vi "read section.vi"(11 "section":string="S1") -> (3 "output cluster":T1)   [LabVIEW 2017, in "GUI.lvlib"]
uses:
  GUI.lvlib
  <vilib>/Utility/config.llb/NI_LVConfig.lvlib
panel:
  in  "PxS":T2
  in  "Px":T3
  in  "Tx":T4
  in  "TxO":T5
  in  "TxA":T6
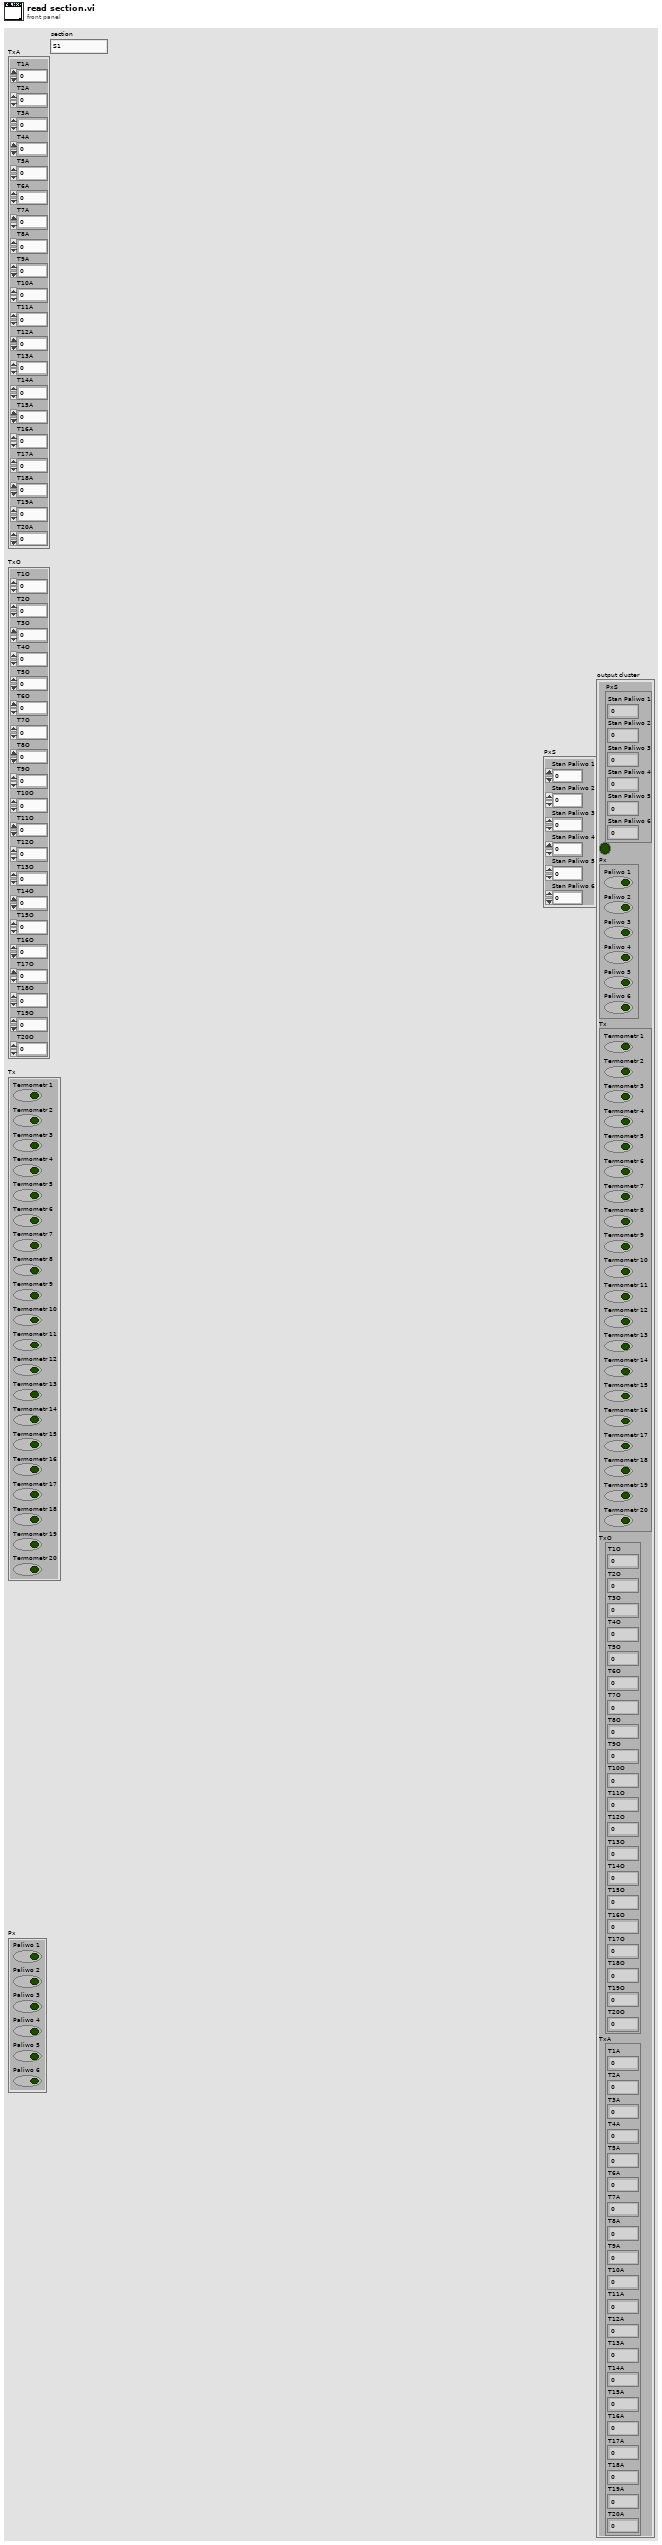
[diagram p1: front panel]
types:
  T1 = cluster{"PxS":cluster{"Stan Paliwo 1":dbl, "Stan Paliwo 2":dbl, "Stan Paliwo 3":dbl, "Stan Paliwo 4":dbl, "Stan Paliwo 5":dbl, "Stan Paliwo 6":dbl}, bool, "Px":cluster{"Paliwo 1":bool, "Paliwo 2":bool, "Paliwo 3":bool, "Paliwo 4":bool, "Paliwo 5":bool, "Paliwo 6":bool}, "Tx":cluster{"Termometr 1":bool, "Termometr 2":bool, "Termometr 3":bool, "Termometr 4":bool, "Termometr 5":bool, "Termometr 6":bool, "Termometr 7":bool, "Termometr 8":bool, "Termometr 9":bool, "Termometr 10":bool, "Termometr 11":bool, "Termometr 12":bool, "Termometr 13":bool, "Termometr 14":bool, "Termometr 15":bool, "Termometr 16":bool, "Termometr 17":bool, "Termometr 18":bool, "Termometr 19":bool, "Termometr 20":bool}, "TxO":cluster{"T1O":dbl, "T2O":dbl, "T3O":dbl, "T4O":dbl, "T5O":dbl, "T6O":dbl, "T7O":dbl, "T8O":dbl, "T9O":dbl, "T10O":dbl, "T11O":dbl, "T12O":dbl, "T13O":dbl, "T14O":dbl, "T15O":dbl, "T16O":dbl, "T17O":dbl, "T18O":dbl, "T19O":dbl, "T20O":dbl}, "TxA":cluster{"T1A":dbl, "T2A":dbl, "T3A":dbl, "T4A":dbl, "T5A":dbl, "T6A":dbl, "T7A":dbl, "T8A":dbl, "T9A":dbl, "T10A":dbl, "T11A":dbl, "T12A":dbl, "T13A":dbl, "T14A":dbl, "T15A":dbl, "T16A":dbl, "T17A":dbl, "T18A":dbl, "T19A":dbl, "T20A":dbl}}
  T2 = cluster{"Stan Paliwo 1":dbl, "Stan Paliwo 2":dbl, "Stan Paliwo 3":dbl, "Stan Paliwo 4":dbl, "Stan Paliwo 5":dbl, "Stan Paliwo 6":dbl}
  T3 = cluster{"Paliwo 1":bool, "Paliwo 2":bool, "Paliwo 3":bool, "Paliwo 4":bool, "Paliwo 5":bool, "Paliwo 6":bool}
  T4 = cluster{"Termometr 1":bool, "Termometr 2":bool, "Termometr 3":bool, "Termometr 4":bool, "Termometr 5":bool, "Termometr 6":bool, "Termometr 7":bool, "Termometr 8":bool, "Termometr 9":bool, "Termometr 10":bool, "Termometr 11":bool, "Termometr 12":bool, "Termometr 13":bool, "Termometr 14":bool, "Termometr 15":bool, "Termometr 16":bool, "Termometr 17":bool, "Termometr 18":bool, "Termometr 19":bool, "Termometr 20":bool}
  T5 = cluster{"T1O":dbl, "T2O":dbl, "T3O":dbl, "T4O":dbl, "T5O":dbl, "T6O":dbl, "T7O":dbl, "T8O":dbl, "T9O":dbl, "T10O":dbl, "T11O":dbl, "T12O":dbl, "T13O":dbl, "T14O":dbl, "T15O":dbl, "T16O":dbl, "T17O":dbl, "T18O":dbl, "T19O":dbl, "T20O":dbl}
  T6 = cluster{"T1A":dbl, "T2A":dbl, "T3A":dbl, "T4A":dbl, "T5A":dbl, "T6A":dbl, "T7A":dbl, "T8A":dbl, "T9A":dbl, "T10A":dbl, "T11A":dbl, "T12A":dbl, "T13A":dbl, "T14A":dbl, "T15A":dbl, "T16A":dbl, "T17A":dbl, "T18A":dbl, "T19A":dbl, "T20A":dbl}
  T7 = typedef "NI_LVConfig.lvlib/Config Data RefNum.ctl" = refnum<k1>
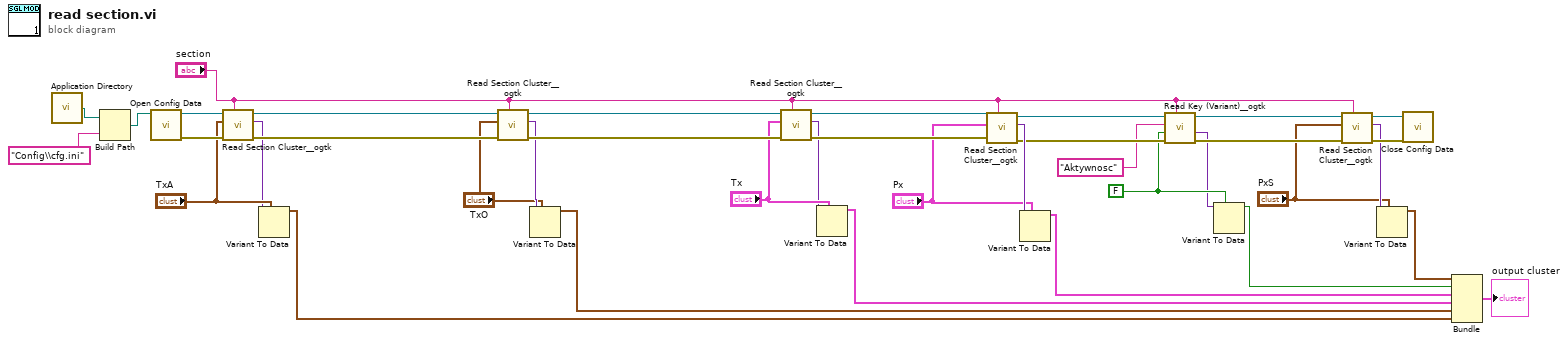
[diagram p0: block diagram]
diagram:
  w11 = FALSE
  n1 = call <vilib>:"Application Directory.vi"() -> ("Application Directory"=w21:path)
  n2 = Build Path(base path=w21, name or relative path="Config\\cfg.ini") -> (appended path=w23:path)
  n3 = call <vilib>:"Open Config Data.vi"("configuration file path"=w23) -> ("error out"=w34:errorcluster, "refnum"=w15:T7)  [unwired: 8 in, 1 out]
  n4 = call <userlib>:"Read Section Cluster__ogtk.vi"("section (optional)"="section", "error in (no error)"=w34, "Section Formatted Cluster Type"="TxA", "refnum"=w15) -> ("error out"=w36:errorcluster, "Section Formatted Cluster"=w26:variant, "dup refnum"=w24:T7)  [unwired: 3 in, 2 out]
  n5 = Variant To Data(type="TxA", Variant=w26) -> (data=w20:T6)  [unwired: 1 in, 1 out]
  n6 = call <userlib>:"Read Section Cluster__ogtk.vi"("section (optional)"="section", "error in (no error)"=w36, "Section Formatted Cluster Type"="TxO", "refnum"=w24) -> ("error out"=w37:errorcluster, "Section Formatted Cluster"=w29:variant, "dup refnum"=w25:T7)  [unwired: 3 in, 2 out]
  n7 = Variant To Data(type="TxO", Variant=w29) -> (data=w19:T5)  [unwired: 1 in, 1 out]
  n8 = call <userlib>:"Read Section Cluster__ogtk.vi"("section (optional)"="section", "error in (no error)"=w37, "Section Formatted Cluster Type"="Tx", "refnum"=w25) -> ("error out"=w35:errorcluster, "Section Formatted Cluster"=w30:variant, "dup refnum"=w16:T7)  [unwired: 3 in, 2 out]
  n9 = Variant To Data(type="Tx", Variant=w30) -> (data=w18:T4)  [unwired: 1 in, 1 out]
  n10 = call <userlib>:"Read Section Cluster__ogtk.vi"("section (optional)"="section", "error in (no error)"=w35, "Section Formatted Cluster Type"="Px", "refnum"=w16) -> ("error out"=w14:errorcluster, "Section Formatted Cluster"=w33:variant, "dup refnum"=w13:T7)  [unwired: 3 in, 2 out]
  n11 = Variant To Data(type="Px", Variant=w33) -> (data=w17:T3)  [unwired: 1 in, 1 out]
  n12 = call <userlib>:"Read Key (Variant)__ogtk.vi"("section"="section", "error in (no error)"=w14, "type"=w11, "key (optional)"="Aktywnosc", "refnum"=w13) -> ("error out"=w38:errorcluster, "key-value"=w10:variant, "refnum out"=w8:T7)  [unwired: 3 in, 1 out]
  n13 = Variant To Data(type=w11, Variant=w10) -> (data=w9:bool)  [unwired: 1 in, 1 out]
  n14 = call <userlib>:"Read Section Cluster__ogtk.vi"("section (optional)"="section", "error in (no error)"=w38, "Section Formatted Cluster Type"="PxS", "refnum"=w8) -> ("error out"=w5:errorcluster, "Section Formatted Cluster"=w4:variant, "dup refnum"=w6:T7)  [unwired: 3 in, 2 out]
  n15 = Variant To Data(type="PxS", Variant=w4) -> (data=w2:T2)  [unwired: 1 in, 1 out]
  n16 = call <vilib>:"Close Config Data.vi"("error in (no error)"=w5, "refnum"=w6) -> ()  [unwired: 8 in, 2 out]
  n17 = Bundle("PxS"=w2, w9, "Px"=w17, "Tx"=w18, "TxO"=w19, "TxA"=w20) -> (→"output cluster":T1)  [unwired: 1 in]
